vi "readbinary.vi"(7 "?":u16(ring) items=["extended precision", "double precision", "single precision", "8 bit byte"], 8 "base path":path, 9 "file index":u64, 10 "data column":string) -> (3 "data":ext[](array[numeric]))   [LabVIEW 2015]
panel:
  in  "?":ext[](array[numeric])
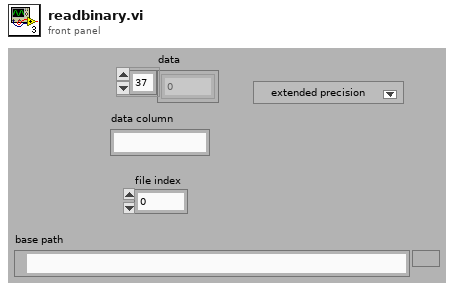
[diagram p1: front panel]
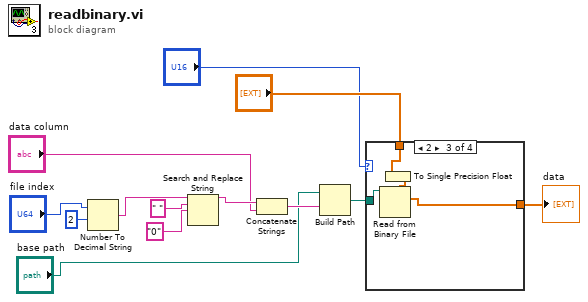
[diagram p0: block diagram]
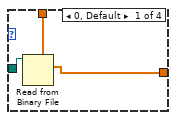
[diagram p2: hidden frame]
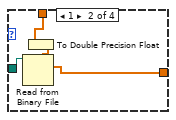
[diagram p3: hidden frame]
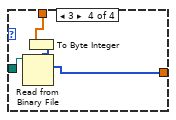
[diagram p4: hidden frame]
diagram:
  n1 = Number To Decimal String(number="file index", width (-)=2) -> (decimal integer string=w10:string)
  n2 = Search and Replace String(input string=w10, search string=" ", replace string="0") -> (result string=w9:string)  [unwired: 2 in, 6 out]
  n3 = Concatenate Strings(w9, "data column") -> (w8:string)
  n4 = Build Path(base path="base path", name or relative path=w8) -> (appended path=w4:path)
  n5 = case shown="2" "?" {
    tunnel: w4 -> [w16 w20 w24 w28]
    tunnel: "?" -> [w15 w19 w23 w27]
    tunnel: [w14 w18 w22 w26] -> w2
    frame 0, Default {
      n6 = Read from Binary File(5:w15, 11:w16) -> (2:w14:ext[])  [unwired: 1 in, 6 out]
    }
    frame 1 {
      n7 = To Double Precision Float(number=w19) -> (double precision float=w17:dbl[])
      n8 = Read from Binary File(5:w17, 11:w20) -> (2:w18:dbl[])  [unwired: 1 in, 6 out]
    }
    frame 2 {
      n9 = To Single Precision Float(number=w23) -> (single precision float=w21:sgl[])
      n10 = Read from Binary File(5:w21, 11:w24) -> (2:w22:sgl[])  [unwired: 1 in, 6 out]
    }
    frame 3 {
      n11 = To Byte Integer(number=w27) -> (8bit integer=w25:i8[])
      n12 = Read from Binary File(5:w25, 11:w28) -> (2:w26:i8[])  [unwired: 1 in, 6 out]
    }
  }
  "data" <- w2
